vi "实时数据参数入列队.vi"(11 "发送实时数据选择框":T1) -> (0 "错误输出":errorcluster)   [LabVIEW 2016]
panel:
  out "数组":string[](array[string])
  # "水样测量数据"
  # "零点核查数据"
  # "跨度核查数据"
  # "加标回收数据"
  # "平行样数据"
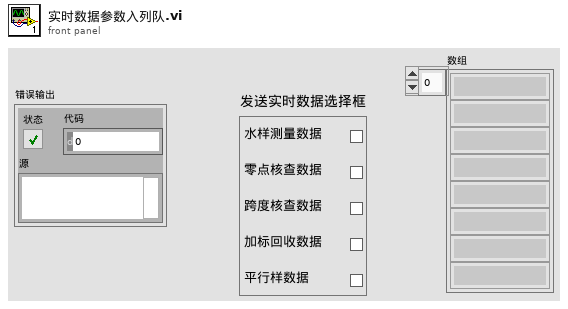
[diagram p1: front panel]
types:
  T1 = cluster{"水样测量数据":bool, "零点核查数据":bool, "跨度核查数据":bool, "加标回收数据":bool, "平行样数据":bool}
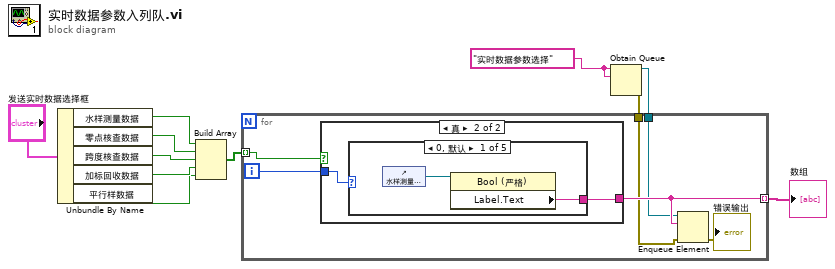
[diagram p0: block diagram]
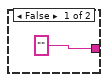
[diagram p2: hidden frame]
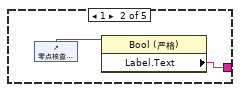
[diagram p3: hidden frame]
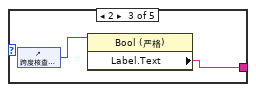
[diagram p4: hidden frame]
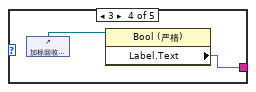
[diagram p5: hidden frame]
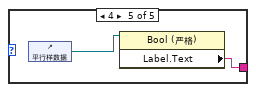
[diagram p6: hidden frame]
diagram:
  w2 = "实时数据参数选择" ("名称（未命名）")
  n1 = Unbundle By Name("发送实时数据选择框") -> ("水样测量数据"=w10:bool, "零点核查数据"=w9:bool, "跨度核查数据"=w8:bool, "加标回收数据"=w7:bool, "平行样数据"=w6:bool)
  n2 = Build Array(w10, w9, w8, w7, w6) -> (w5:bool[])
  n3 = Obtain Queue(name (unnamed)=w2, element data type=w2) -> (queue out=w3:refnum<queue>, error out=w1:errorcluster)  [unwired: 3 in, 1 out]
  n4 = for {
    tunnel: w5 -> [w17] mode=indexing
    tunnel: [w15] -> w4 mode=indexing
    tunnel: w3 -> [w14]
    tunnel: w1 -> [w13]
    i -> [w16]
    n5 = case shown="真" w17 {
      tunnel: w16 -> [_ w20]
      tunnel: ["" ("Label.Text") w19] -> w15
      frame False {
      }
      frame True {
        n6 = case shown="0, 默认" w20 {
          tunnel: [w21 w23 w26 w27 w29] -> w19
          frame 0, Default {
            n7 = control-ref of="水样测量数据"() -> (w22:refnum<vi>)
            n8 = property class="Bool (严格)"(reference=w22) -> ("Label.Text"=w21:string)  [unwired: 1 in, 2 out]
          }
          frame 1 {
            n9 = control-ref of="零点核查数据"() -> (w24:refnum<vi>)
            n10 = property class="Bool (严格)"(reference=w24) -> ("Label.Text"=w23:string)  [unwired: 1 in, 2 out]
          }
          frame 2 {
            n11 = control-ref of="跨度核查数据"() -> (w25:refnum<vi>)
            n12 = property class="Bool (严格)"(reference=w25) -> ("Label.Text"=w26:string)  [unwired: 1 in, 2 out]
          }
          frame 3 {
            n13 = control-ref of="加标回收数据"() -> (w28:refnum<vi>)
            n14 = property class="Bool (严格)"(reference=w28) -> ("Label.Text"=w27:string)  [unwired: 1 in, 2 out]
          }
          frame 4 {
            n15 = control-ref of="平行样数据"() -> (w30:refnum<vi>)
            n16 = property class="Bool (严格)"(reference=w30) -> ("Label.Text"=w29:string)  [unwired: 1 in, 2 out]
          }
        }
      }
    }
    n17 = Enqueue Element(queue=w14, element=w15, error in (no error)=w13) -> (error out=→"错误输出":errorcluster)  [unwired: 1 in, 2 out]
  }
  "数组" <- w4
